vi "preprocess_shader.vi"(1 "Shader In":string) -> (0 "Shader Out":string)   [LabVIEW 2019]
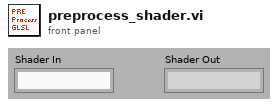
[diagram p1: front panel]
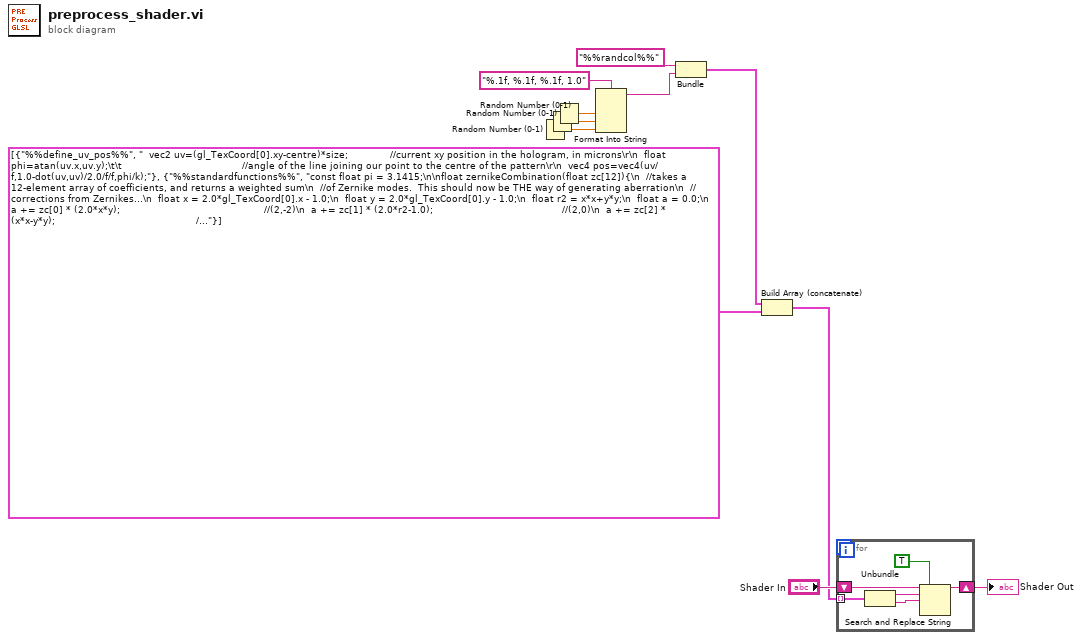
[diagram p0: block diagram]
diagram:
  n1 = Random Number (0-1)() -> (number: 0 to 1=w1:dbl)
  n2 = Random Number (0-1)() -> (number: 0 to 1=w2:dbl)
  n3 = Random Number (0-1)() -> (number: 0 to 1=w3:dbl)
  n4 = Format Into String(format string="%.1f, %.1f, %.1f, 1.0", w3, w2, w1) -> (resulting string=w5:string)  [unwired: 2 in, 1 out]
  n5 = Bundle("%%randcol%%", w5) -> (w7:cluster{string, string})  [unwired: 1 in]
  n6 = Build Array (concatenate)(w7, cluster{string, string}[] [{"%%define_uv_pos%%", "  vec2 uv=(gl_TexCoord[0].xy-centre)*size;              //current xy position in the hologram, in microns\r\n  float phi=atan(uv.x,uv.y);\t\t                                        //angle of the line joining our point to the centre of the pattern\r\n  vec4 pos=vec4(uv/f,1.0-dot(uv,uv)/2.0/f/f,phi/k);"}, {"%%standardfunctions%%", "const float pi = 3.1415;\n\nfloat zernikeCombination(float zc[12]){\n  //takes a 12-element array of coefficients, and returns a weighted sum\n  //of Zernike modes.  This should now be THE way of generating aberration\n  //corrections from Zernikes...\n  float x = 2.0*gl_TexCoord[0].x - 1.0;\n  float y = 2.0*gl_TexCoord[0].y - 1.0;\n  float r2 = x*x+y*y;\n  float a = 0.0;\n  a += zc[0] * (2.0*x*y);                                                //(2,-2)\n  a += zc[1] * (2.0*r2-1.0);                                           //(2,0)\n  a += zc[2] * (x*x-y*y);                                               //(2,2)\n  a += zc[3] * (3.0*x*x*y-y*y*y);                                 //(3,-3)\n  a += zc[4] * ((3.0*r2-2.0)*y);                                    //(3,-1)\n  a += zc[5] * ((3.0*r2-2.0)*x);                                    //(3,1)\n  a += zc[6] * (x*x*x-3.0*x*y*y);                                 //(3,3)\n  a += zc[7] * (4.0*x*y*(x*x-y*y));                              //(4,-4)\n  a += zc[8] * ((4.0*r2-3.0)*2.0*x*y);                          //(4,-2)\n  a += zc[9] * (6.0*r2*r2-6*r2+1);                               //(4,0)\n  a += zc[10] * ((4.0*r2-3.0)*(x*x-y*y));                      //(4,2)\n  a += zc[11] * (x*x*x*x-6.0*x*x*y*y+y*y*y*y);          //(4,4)\n  return a;\n}\n\n\nfloat zernikeAberration(){\n//this function is exactly the same as zernikeCombination, except that it uses a uniform\n//called zernikeCoefficients as its argument.  This avoids copying the array = more efficient.\n  //takes a 12-element array of coefficients, and returns a weighted sum\n  //of Zernike modes.  This should now be THE way of generating aberration\n  //corrections from Zernikes...\n  float x = 2.0*gl_TexCoord[0].x - 1.0;\n  float y = 2.0*gl_TexCoord[0].y - 1.0;\n  float r2 = x*x+y*y;\n  float a = 0.0;\n  a += zernikeCoefficients[0] * (2.0*x*y);                                                //(2,-2)\n  a += zernikeCoefficients[1] * (2.0*r2-1.0);                                           //(2,0)\n  a += zernikeCoefficients[2] * (x*x-y*y);                                               //(2,2)\n  a += zernikeCoefficients[3] * (3.0*x*x*y-y*y*y);                                 //(3,-3)\n  a += zernikeCoefficients[4] * ((3.0*r2-2.0)*y);                                    //(3,-1)\n  a += zernikeCoefficients[5] * ((3.0*r2-2.0)*x);                                    //(3,1)\n  a += zernikeCoefficients[6] * (x*x*x-3.0*x*y*y);                                 //(3,3)\n  a += zernikeCoefficients[7] * (4.0*x*y*(x*x-y*y));                              //(4,-4)\n  a += zernikeCoefficients[8] * ((4.0*r2-3.0)*2.0*x*y);                          //(4,-2)\n  a += zernikeCoefficients[9] * (6.0*r2*r2-6*r2+1);                               //(4,0)\n  a += zernikeCoefficients[10] * ((4.0*r2-3.0)*(x*x-y*y));                      //(4,2)\n  a += zernikeCoefficients[11] * (x*x*x*x-6.0*x*x*y*y+y*y*y*y);          //(4,4)\n  return a;\n}\n\nfloat wrap2pi(float phase){\n  return mod(phase + pi, 2*pi) -pi;\n}\n\nfloat phase_to_gray(float phase){\n  return phase/2.0/pi +0.5;\n}\n\nvec2 unitvector(float angle){\n  return vec2(cos(angle), sin(angle));\n}\n\nfloat apply_LUT(float phase){\n  int phint = int(floor((phase/2.0/pi +0.5)*30.9999999)); //blazing table element just before our point\r\n  float alpha = fract((phase/2.0/pi +0.5)*30.9999999); //remainder\r\n  return mix(blazing[phint], blazing[phint+1], alpha); //this uses the blazing table with linear interpolation\n}\n\nvec4 gray_to_16bit(float gray){\n  return vec4(fract(gray * 255.9999), floor(gray * 255.9999)/255.0, 0.0, 1.0);\n}"}]) -> (w8:cluster{string, string}[])
  n7 = for {
    tunnel: w8 -> [w16] mode=indexing
    shift-right: [w12] -> w9
    shift-left: "Shader In" -> [w17]
    n8 = Unbundle(w16) -> (w15:string, w14:string)
    n9 = Search and Replace String(replace all?=TRUE ("replace all? (F)"), input string=w17, search string=w15, replace string=w14) -> (result string=w12:string)  [unwired: 4 in, 3 out]
  }
  "Shader Out" <- w9
